vi "Sequence-Load.vi"(8 "error in (no error)":errorcluster, 10 "Sequence String":string, 11 "MCListbox Refnum":refnum<vi>) -> (0 "error out":errorcluster, 3 "MCListbox Refnum(dup)":refnum<vi>)   [LabVIEW 2020, in "CSMScript-Engine(Lite).lvlib"]
uses:
  CSMScript-Engine(Lite).lvlib
  <userlib>/_NEVSTOP/Communicable State Machine(CSM)/Communicable State Machine.lvlib
panel:
  # "Connector Pane"
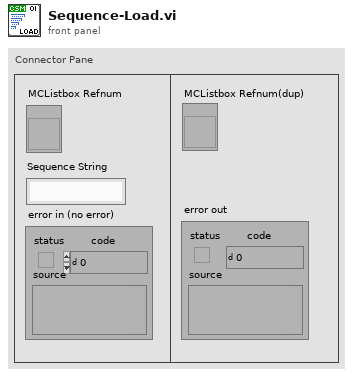
[diagram p1: front panel]
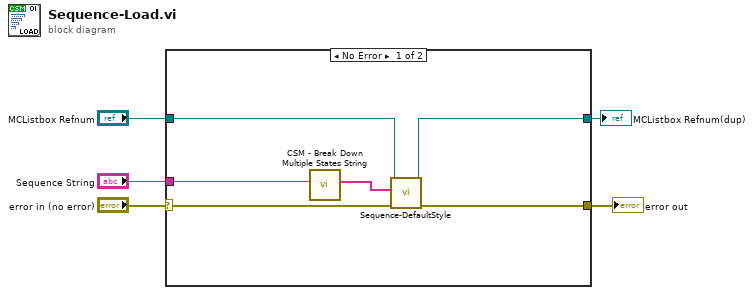
[diagram p0: block diagram]
diagram:
  n1 = case shown="No Error" "error in (no error)" {
    selector: "error in (no error)" -> [w6 w13]
    tunnel: [w7 w13] -> w5
    tunnel: "MCListbox Refnum" -> [w10 w12]
    tunnel: [w8 w12] -> w2
    tunnel: "Sequence String" -> [w11 _]
    frame No Error {
      n2 = call <userlib>:"CSM - Break Down Multiple States String.vi"("States"=w11) -> ("Multiple States"=w9:string[])  [unwired: 10 in]
      n3 = call "Sequence-DefaultStyle.vi"("error in (no error)"=w6, "Test Steps"=w9, "MCListbox Refnum"=w10) -> ("error out"=w7:errorcluster, "MCListbox Refnum(dup)"=w8:refnum<vi>)  [unwired: 7 in]
    }
    frame Error {
    }
  }
  "error out" <- w5
  "MCListbox Refnum(dup)" <- w2
